vi "data-collection.vi"(6 "Time has Elapsed":bool, 9 "Enable Data Collection\n(Excel Spreadsheet)":bool caption="Enable", 10 "Dynamic Data":dynamicdata(waveform), 11 "appended path":path) -> ()   [LabVIEW 2025]
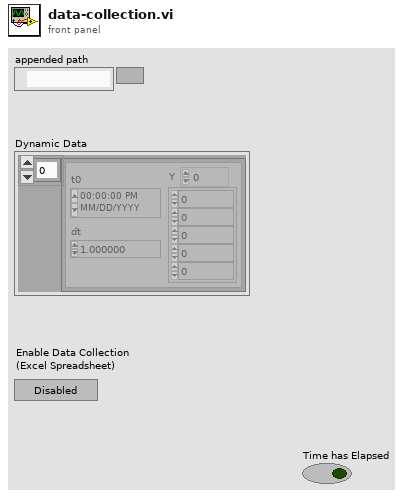
[diagram p1: front panel]
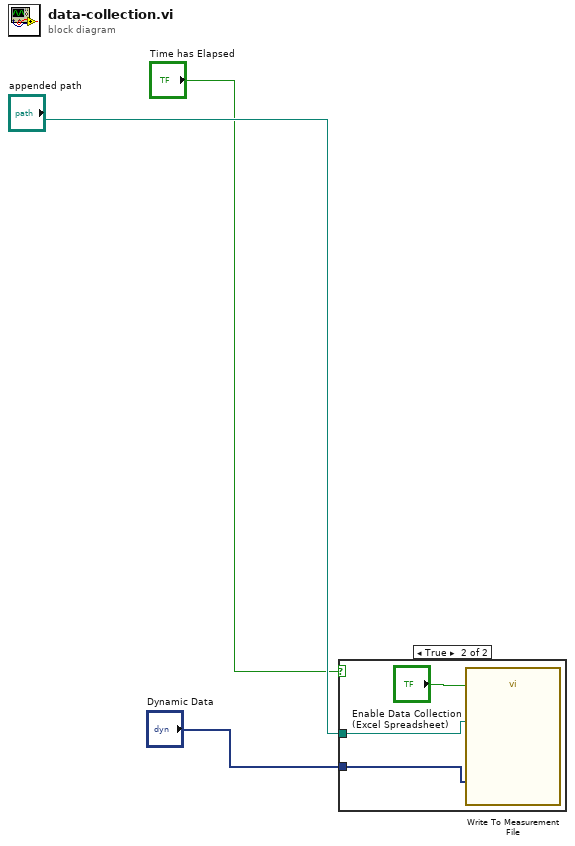
[diagram p0: block diagram]
diagram:
  n1 = case shown="True" "Time has Elapsed" {
    tunnel: "Dynamic Data" -> [_ w6]
    tunnel: "appended path" -> [_ w5]
    frame False {
    }
    frame True {
      n2 = call "Write To Measurement File"("Signals"=w6, "Enable"="Enable Data Collection\n(Excel Spreadsheet)", "Filename"=w5) -> ()  [unwired: 14 in, 3 out]
    }
  }
